vi "CLD 12 Timer.vi"(8 "Fehler (Eingang)":T1, 10 "Zielzeit (s)":dbl, 11 "CLD 12 - Timer-Enum":T2) -> (0 "Fehler (Ausgang)":T1, 2 "Ist Zeit verstrichen?":bool, 3 "Verstrichene Zeit (s,ms)":dbl)   [LabVIEW 2014]
doc: "CLD-Übung 12\n\nDieses VI wird als FGV verwendet. Der Case \"Timer zurücksetzen\" verwendet die aktuelle Zielzeit. Der Case \"Timer starten\" liest eine neue Zielzeit vom Aufrufer aus.\n\n\n\n\n\nHinweise zum Auslesen der Zeit während der Pause: Der Entwickler sollte die Funktion \"Zeit lesen\" nicht während der Pause aufrufen. Mit Hilfe einer Case-Struktur kann \"Status abfragen\" jedoch präventiv für diese Möglichkeit programmiert werden."
uses:
  CLD12 Timer Enum.ctl
panel:
  out "Verstrichene Zeit (s)":dbl
  out "Verstrichene Zeit (s,sssss)":dbl
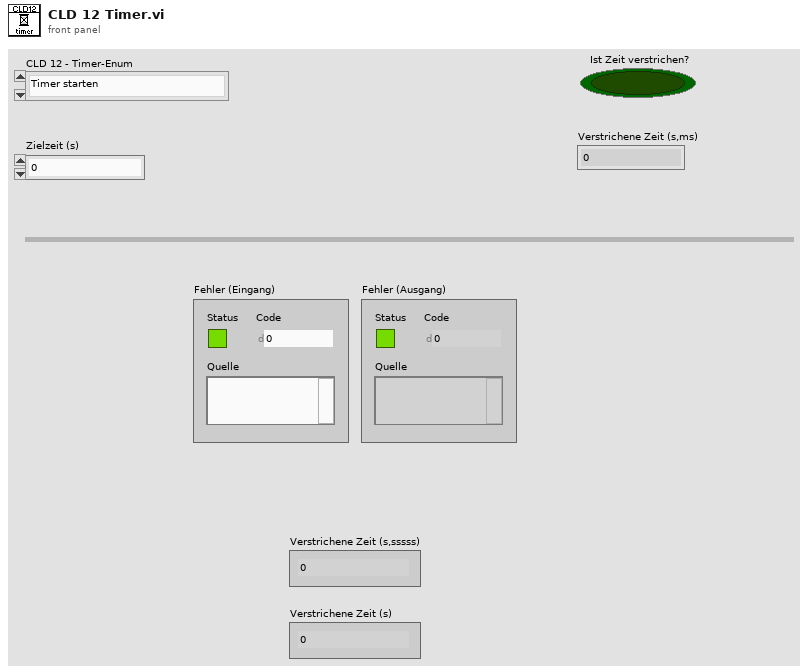
[diagram p1: front panel]
types:
  T1 = cluster{"Status":bool, "Code":i32, "Quelle":string}
  T2 = typedef "CLD12 Timer Enum.ctl" = enum16{"Timer starten", "Zeit lesen", "Anhalten", "Fortsetzen", "Timer zurücksetzen"}
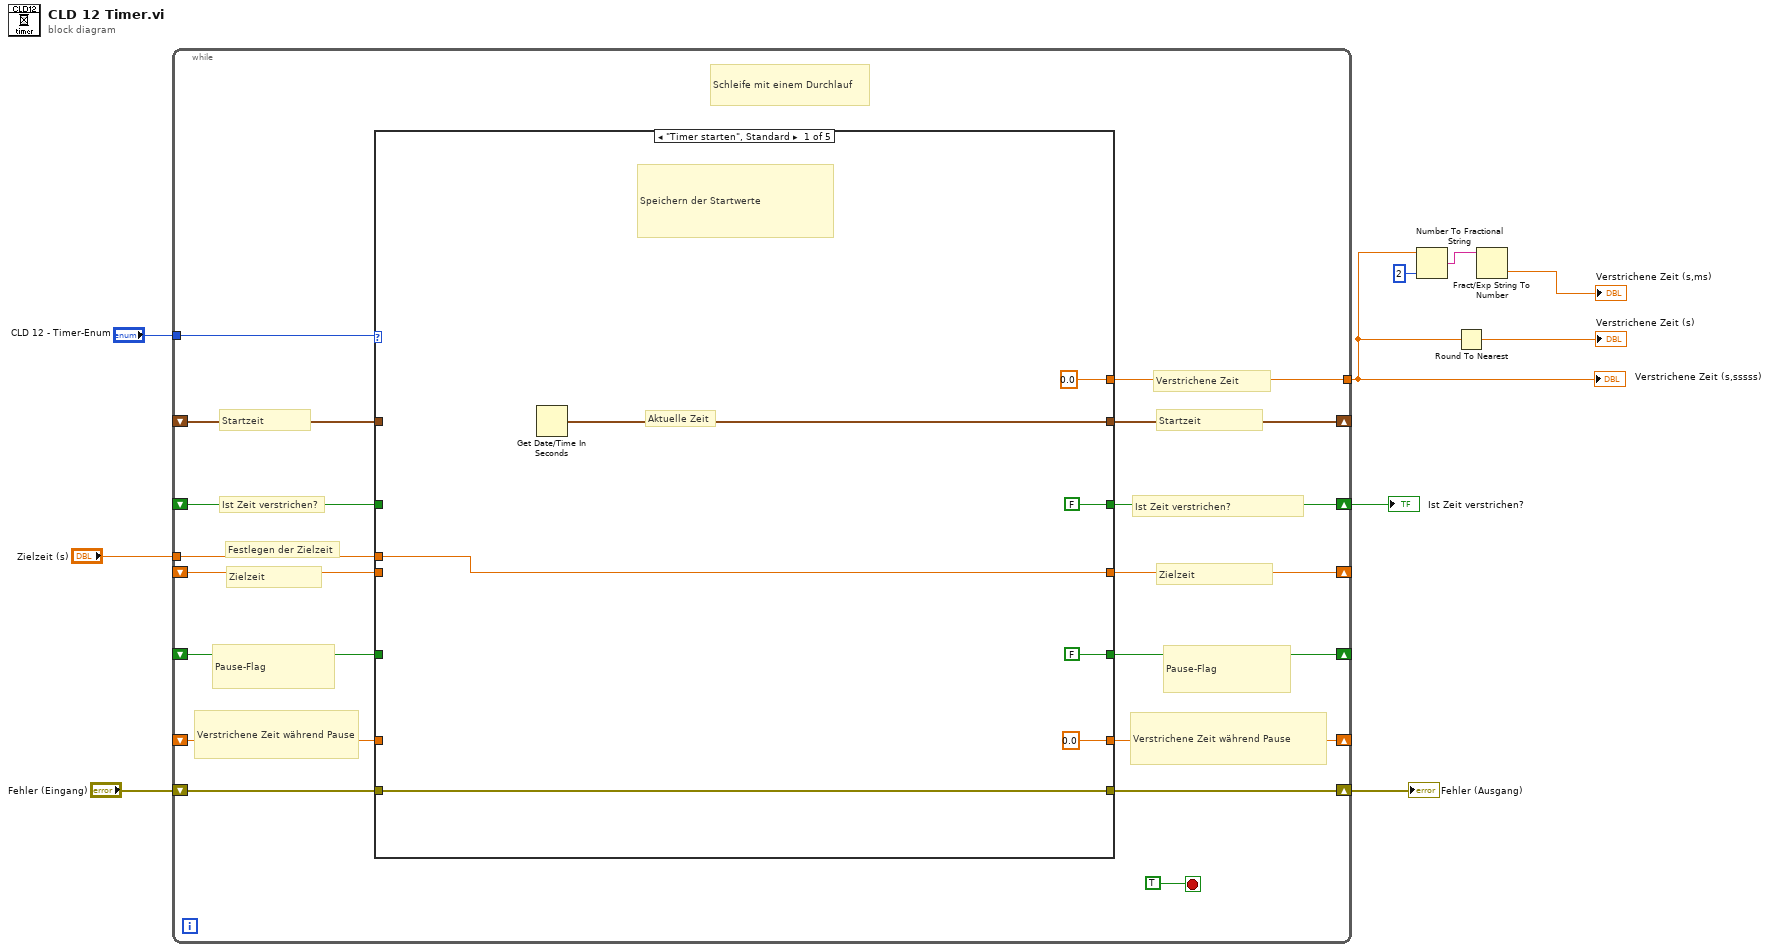
[diagram p0: block diagram]
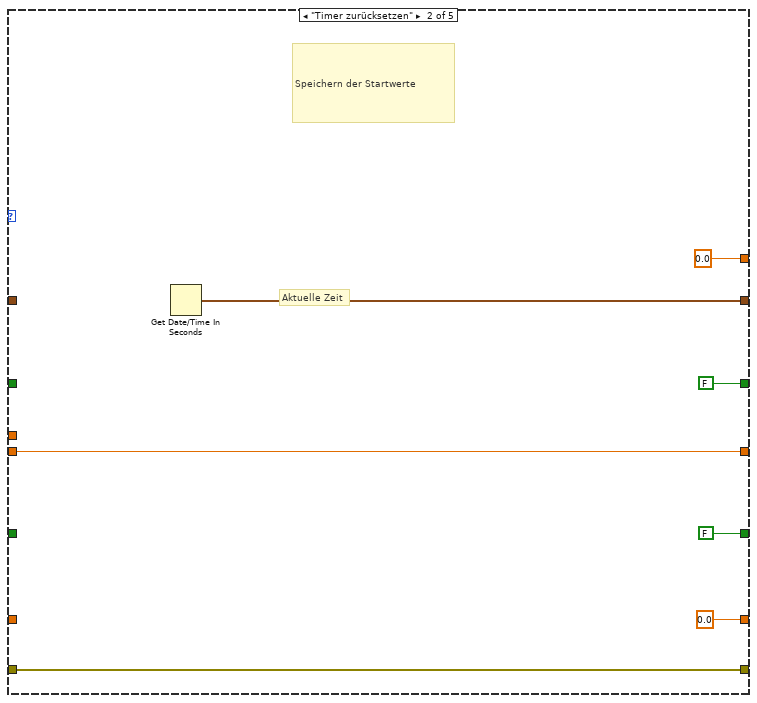
[diagram p2: hidden frame]
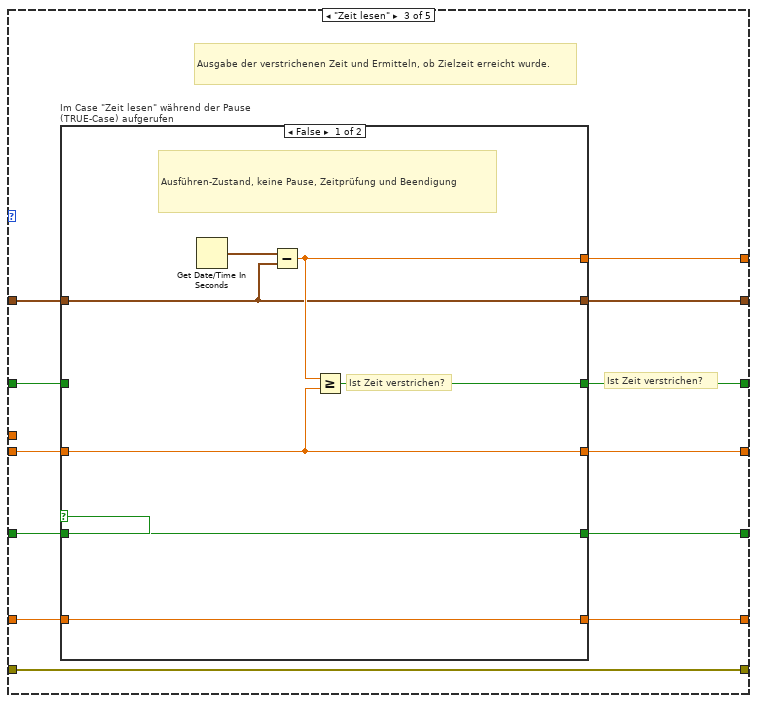
[diagram p3: hidden frame]
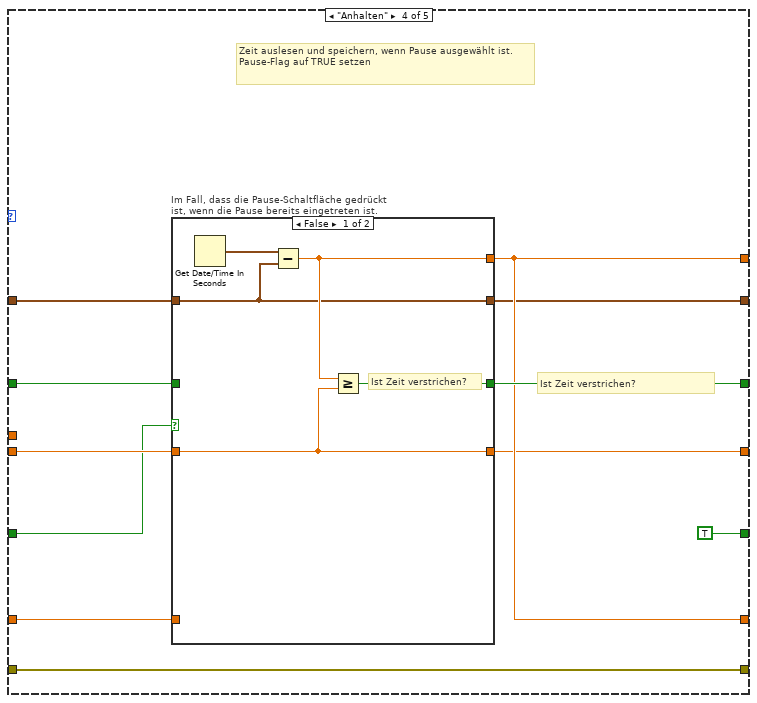
[diagram p5: hidden frame]
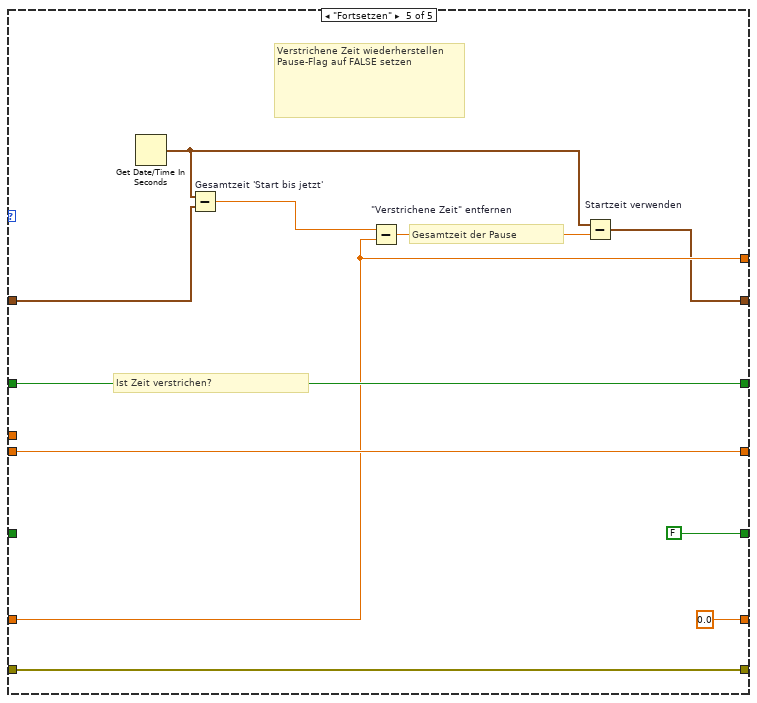
[diagram p7: hidden frame]
diagram:
  n1 = while {
    tunnel: "CLD 12 - Timer-Enum" -> [w26]
    shift-right: [w24] -> _
    shift-left: _ -> [w23]
    tunnel: [w22] -> w4
    shift-right: [w21] -> w9
    shift-left: "Fehler (Eingang)" -> [w20]
    tunnel: "Zielzeit (s)" -> [w17]
    shift-right: [w18] -> _
    shift-left: _ -> [w19]
    shift-right: [w16] -> w6
    shift-left: _ -> [w15]
    shift-right: [w14] -> _
    shift-left: _ -> [w13]
    shift-right: [w12] -> _
    shift-left: _ -> [w11]
    stop <- TRUE ("Stopp") stop-if-true
    # "Startzeit"
    # "Startzeit"
    # "Verstrichene Zeit"
    # "Zielzeit"
    # "Zielzeit"
    # "Festlegen der Zielzeit"
    # "Ist Zeit verstrichen?"
    # "Ist Zeit verstrichen?"
    # "Pause-Flag"
    # "Pause-Flag"
    # "Verstrichene Zeit während Pause"
    # "Verstrichene Zeit während Pause"
    # "Schleife mit einem Durchlauf"
    n2 = case shown="\"Timer starten\", Standard" w26 {
      tunnel: [w33 w40 w44 w64 w84] -> w24
      tunnel: w23 -> [_ _ w51 w74 w89]
      tunnel: [0.0 ("Verstrichene Zeit") 0.0 ("Verstrichene Zeit") w47 w69 w87] -> w22
      tunnel: [w31 w38 w50 w73 w94] -> w21
      tunnel: w20 -> [w31 w38 w50 w73 w94]
      tunnel: w19 -> [_ w34 w49 w72 w93]
      tunnel: [w27 w34 w49 w65 w93] -> w18
      tunnel: w17 -> [w27 _ _ _ _]
      tunnel: [FALSE FALSE w48 w71 w91] -> w16
      tunnel: w15 -> [_ _ w41 w68 w91]
      tunnel: [FALSE FALSE w43 TRUE FALSE] -> w14
      tunnel: w13 -> [_ _ w42 w67 _]
      tunnel: [0.0 0.0 w45 w69 0.0] -> w12
      tunnel: w11 -> [_ _ w46 w66 w87]
      frame "Timer starten", Default {
        # "Aktuelle Zeit"
        # "Speichern der Startwerte"
        n3 = Get Date/Time In Seconds() -> (seconds since 1Jan1904=w33:timestamp)
      }
      frame "Timer zurücksetzen" {
        # "Aktuelle Zeit"
        # "Speichern der Startwerte"
        n4 = Get Date/Time In Seconds() -> (seconds since 1Jan1904=w40:timestamp)
      }
      frame "Zeit lesen" {
        # "Ist Zeit verstrichen?"
        # "Ausgabe der verstrichenen Zeit und Ermitteln, ob Zielzeit erreicht wurde."
        n5 = case "Im Case \"Zeit lesen\" während der Pause (TRUE-Case) aufgerufen" shown="False" w42 {
          tunnel: w51 -> [w55 w63]
          tunnel: w49 -> [w54 w62]
          tunnel: [w57 w60] -> w48
          tunnel: [w56 w59] -> w47
          tunnel: w46 -> [w52 w59]
          tunnel: [w52 w59] -> w45
          tunnel: [w55 w63] -> w44
          tunnel: [w54 w62] -> _
          tunnel: [w53 w61] -> w43
          tunnel: w42 -> [w53 w61]
          tunnel: w41 -> [_ w60]
          frame False {
            # "Ist Zeit verstrichen?"
            # "Ausführen-Zustand, keine Pause, Zeitprüfung und Beendigung"
            n6 = Get Date/Time In Seconds() -> (seconds since 1Jan1904=w58:timestamp)
            n7 = Subtract(x=w58, y=w55) -> (x-y=w56:dbl)
            n8 = Greater Or Equal?(x=w56, y=w54) -> (x >= y?=w57:bool)
          }
          frame True {
            # "Pause-Zustand, nur Ausgabe von Schieberegistern. \"Zeit lesen\" nicht während der Pause aufrufen."
          }
        }
      }
      frame "Anhalten" {
        # "Ist Zeit verstrichen?"
        # "Zeit auslesen und speichern, wenn Pause ausgewählt ist.\nPause-Flag auf TRUE setzen"
        n9 = case "Im Fall, dass die Pause-Schaltfläche gedrückt ist, wenn die Pause bereits eingetreten ist." shown="False" w67 {
          tunnel: w74 -> [w75 w80]
          tunnel: w72 -> [w76 w81]
          tunnel: [w78 w83] -> w71
          tunnel: [w77 w82] -> w69
          tunnel: w68 -> [_ w83]
          tunnel: w66 -> [_ w82]
          tunnel: [w76 w81] -> w65
          tunnel: [w75 w80] -> w64
          frame False {
            # "Ist Zeit verstrichen?"
            n10 = Get Date/Time In Seconds() -> (seconds since 1Jan1904=w79:timestamp)
            n11 = Subtract(x=w79, y=w75) -> (x-y=w77:dbl)
            n12 = Greater Or Equal?(x=w77, y=w76) -> (x >= y?=w78:bool)
          }
          frame True {
            # "Pause wurde während der Pause aufgerufen.\n\nNur Schieberegister auslesen und Werte weitergeben."
          }
        }
      }
      frame "Fortsetzen" {
        # "Ist Zeit verstrichen?"
        # "Gesamtzeit der Pause"
        # "Verstrichene Zeit wiederherstellen\nPause-Flag auf FALSE setzen"
        n13 = Get Date/Time In Seconds() -> (seconds since 1Jan1904=w86:timestamp)
        n14 = Subtract "Gesamtzeit 'Start bis jetzt'"(x=w86, y=w89) -> (x-y=w88:dbl)
        n15 = Subtract "\"Verstrichene Zeit\" entfernen"(x=w88, y=w87) -> (x-y=w85:dbl)
        n16 = Subtract "Startzeit verwenden"(x=w86, y=w85) -> (x-y=w84:timestamp)
      }
    }
  }
  "Verstrichene Zeit (s,sssss)" <- w4
  "Fehler (Ausgang)" <- w9
  "Ist Zeit verstrichen?" <- w6
  n17 = Number To Fractional String(number=w4, precision (6)=i16 2 ("Genauigkeit (6)")) -> (F-format string=w3:string)  [unwired: 2 in]
  n18 = Round To Nearest(number=w4) -> (nearest integer value=→"Verstrichene Zeit (s)":dbl)
  n19 = Fract/Exp String To Number(string=w3) -> (number=→"Verstrichene Zeit (s,ms)":dbl)  [unwired: 3 in, 1 out]
